vi "REPORT_CMPNT_prepare_header_for_csv.vi"(11 "REPORT_CMPNT_all_info":T1) -> (3 "report_header":string[][](array[string]))   [LabVIEW 2019]
uses:
  typedef/REPORT_CMPNT_all_info.ctl
  _misc/AULocalize/SubVIs/Get Localized Phrase Compact Interface 1D.vi
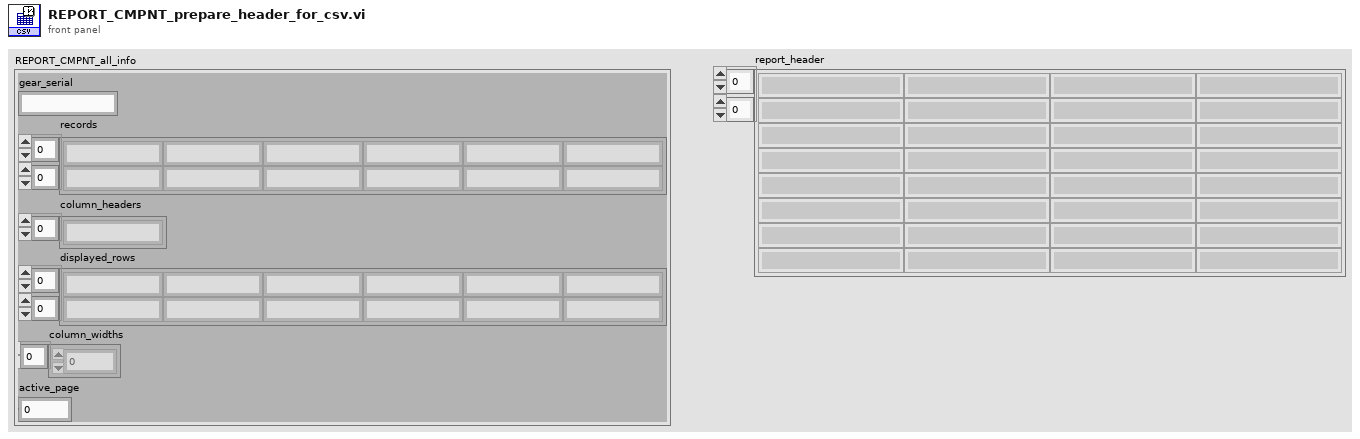
[diagram p1: front panel]
types:
  T1 = typedef "REPORT_CMPNT_all_info.ctl" = cluster{"gear_serial":string, "records":string[][], "column_headers":string[], "displayed_rows":string[][], "column_widths":i16[], "active_page":i32}
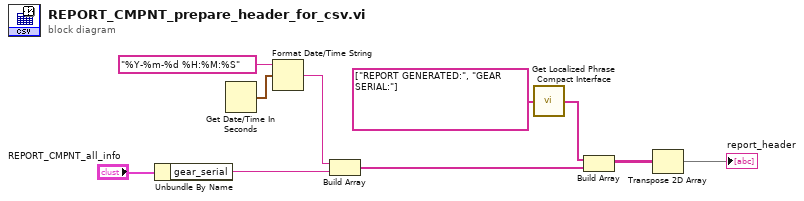
[diagram p0: block diagram]
diagram:
  n1 = Unbundle By Name("REPORT_CMPNT_all_info") -> ("gear_serial"=w2:string)
  n2 = Get Date/Time In Seconds() -> (seconds since 1Jan1904=w9:timestamp)
  n3 = Format Date/Time String(time format string (%c)="%Y-%m-%d %H:%M:%S", seconds (now)=w9) -> (date/time string=w3:string)  [unwired: 1 in]
  n4 = Build Array(w3, w2) -> (w4:string[])
  n5 = call-poly "Get Localized Phrase Compact Interface.vi"("Key"=string[] ["REPORT GENERATED:", "GEAR SERIAL:"]) -> ("Translated Phrase"=w1:string[])
  n6 = Build Array(w1, w4) -> (w7:string[][])
  n7 = Transpose 2D Array(2D array=w7) -> (transposed array=→"report_header":string[][])
